vi "ProgBar_UI.vi"() -> ()   [LabVIEW 2020]
doc: ",,,,,,,,,,,,,,,,,,,,,,,,,,,,,,,,,,,,,,,,,,,,,,,,,,,,,,,,,,,,,,,,,,,,,,,,,,,,,,,,,,,,,,,,,,,,,,,,,,,,,,,,,,,,,,,,,,,,,,,,,,,,,,,,,,,,,,,,,,,,,,,,"
uses:
  controls/ProgBar_Element.ctl
  controls/System_Custom/Cancel.ctl
  controls/ProgBar_Msg.ctl
  <vilib>/Utility/miscctls.llb/LVRectTypeDef.ctl
  <vilib>/Utility/miscctls.llb/LVPositionTypeDef.ctl
panel:
  out "Current_Prgrs":T3(array[cluster]) {"ProgBar_El"."Curr Digital" format="%#_7g"; "ProgBar_El"."Slide Value" scale=0.0..100.0}
  in  "Display":T1[](array[typedef]) {"Curr Digital" format="%#_7g"; "Slide Value" scale=0.0..100.0}
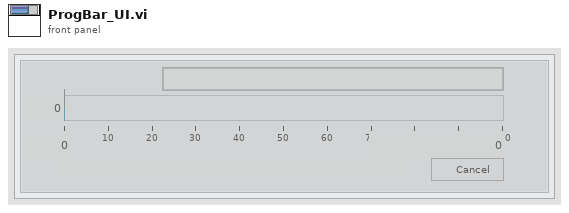
[diagram p1: front panel]
types:
  T1 = typedef "ProgBar_Element.ctl" = cluster{"Label":string, "Slide Value":i32, "Max":dbl, "Curr Digital":dbl, "Min":dbl, "State Info":string, "Cancel":T2}
  T2 = typedef "Cancel.ctl" = bool
  T3 = cluster{"Progress Queue Name":string, "ProgBar_El":T1}[]
  T4 = typedef "ProgBar_Msg.ctl" = cluster{"Que_Name":string, "Label":string, "Max Number of Iterations":i32, "Current Iteration ":i32, "State Info(Optional)":string, "Stop":bool}
  T5 = enum32{"Invalid", "Default", "Floating", "Floating/Auto-Hide", "Modal"}
  T6 = typedef "LVPositionTypeDef.ctl" = cluster{"Left":i32, "Top":i32}
  T7 = typedef "LVRectTypeDef.ctl" = cluster{"Left":i16, "Top":i16, "Right":i16, "Bottom":i16}
  T8 = typedef "LVBoundsTypeDef.ctl" = cluster{"Width":u32, "Height":u32}
  T9 = cluster{"Label":bool, "Slide Value":bool, "Max":bool, "Curr Digital":bool, "Min":bool, "State Info":bool, "Cancel":T2}[]
  T10 = cluster{"Progress Queue Name":string, "ProgBar_El":T1}
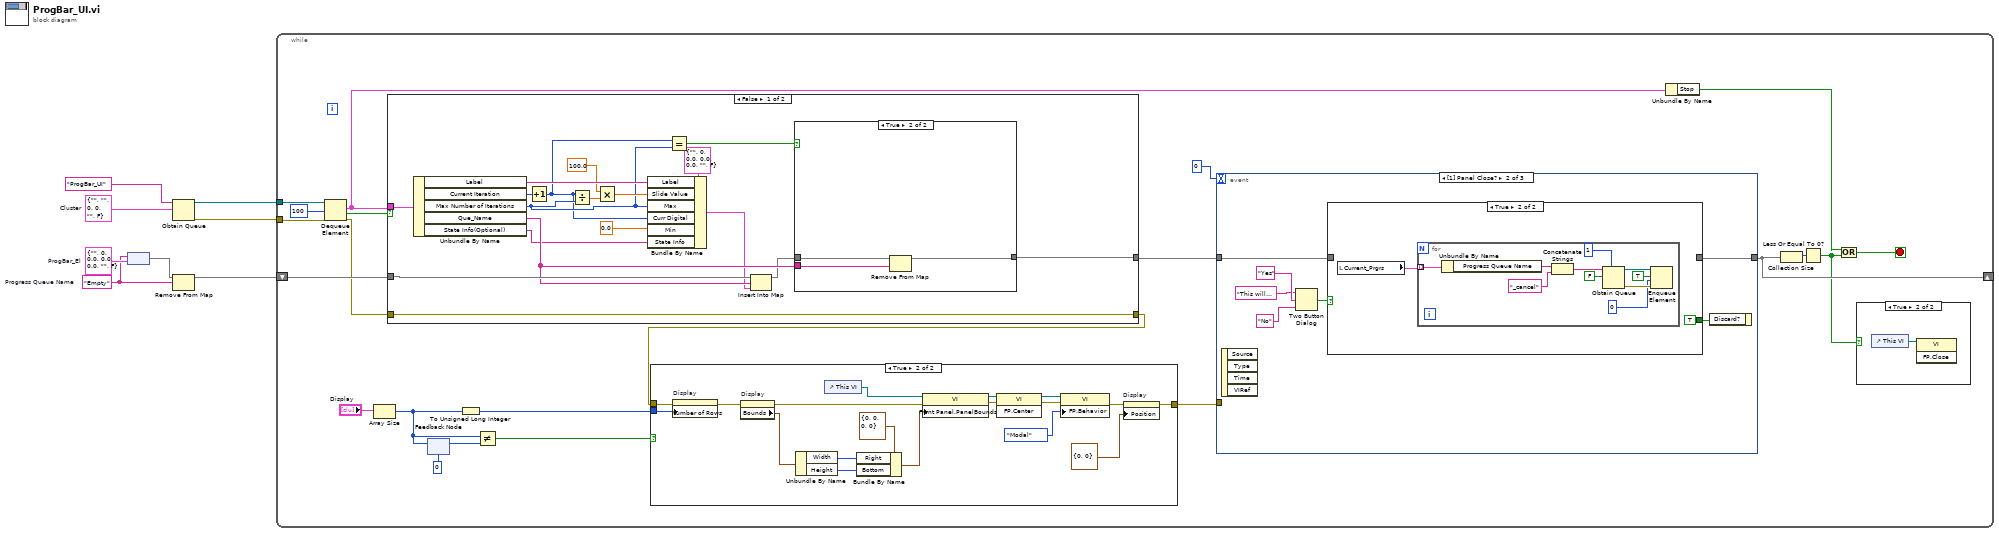
[diagram p0: block diagram]
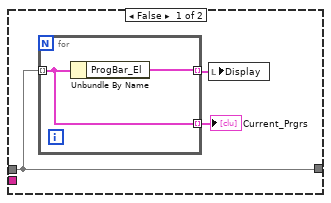
[diagram p2: hidden frame]
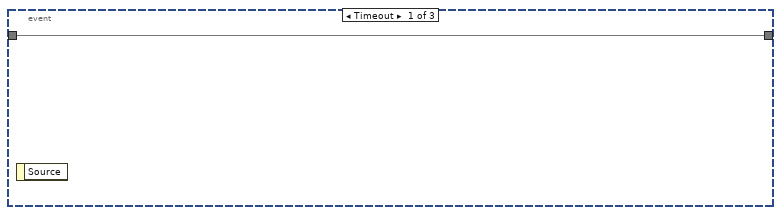
[diagram p5: hidden frame]
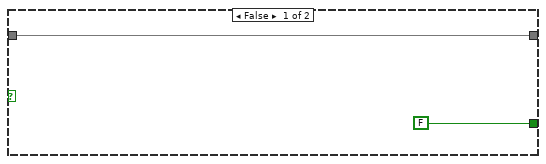
[diagram p6: hidden frame]
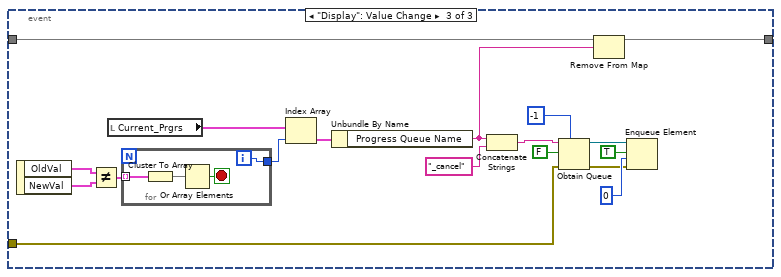
[diagram p7: hidden frame]
diagram:
  w6 = "Empty"  # Progress Queue Name
  w7 = T1 {"Label"="", "Slide Value"=0, "Max"=0.0, "Curr Digital"=0.0, "Min"=0.0, "State Info"="", "Cancel"=FALSE}  # ProgBar_El
  w4 = T4 {"Que_Name"="", "Label"="", "Max Number of Iterations"=0, "Current Iteration "=0, "State Info(Optional)"="", "Stop"=FALSE}  # Cluster
  n1 = node(w6, w7) -> (w5:map{string, T1})
  n2 = Obtain Queue(name (unnamed)="ProgBar_UI" ("Progress Queue Name"), element data type=w4) -> (queue out=w1:refnum<queue>, error out=w2:errorcluster)  [unwired: 3 in, 1 out]
  n3 = Remove From Map(10:w6, 11:w5) -> (3:w3:map{string, T1})  [unwired: 2 out]
  n4 = while {
    tunnel: w1 -> [w30]
    shift-right: [w17] -> _
    shift-left: w3 -> [w29]
    tunnel: w2 -> [w22]
    stop <- w10 stop-if-true
    n5 = Dequeue Element(queue=w30, timeout in ms (-1)=100, error in (no error)=w22) -> (element=w12:T4, timed out?=w25:bool, error out=w24:errorcluster)  [unwired: 1 out]
    n6 = Array Size(array="Display") -> (size(s)=w15:i32)
    n7 = case shown="False" w25 {
      tunnel: w12 -> [w48 _]
      tunnel: w29 -> [w45 w58]
      tunnel: [w35 w58] -> w16
      tunnel: [w44 w57] -> w14
      tunnel: w24 -> [w44 w57]
      frame False {
        n8 = Unbundle By Name(w48) -> ("Label"=w46:string, "Current Iteration"=w32:i32, "Max Number of Iterations"=w33:i32, "Que_Name"=w38:string, "State Info(Optional)"=w37:string)
        n9 = Increment(x=w32) -> (x+1=w31:i32)
        n10 = Divide(x=w31, y=w33) -> (x/y=w41:dbl)
        n11 = Multiply(x=100.0 ("y"), y=w41) -> (x*y=w40:dbl)
        n12 = Bundle By Name(cluster=T1 {"Label"="", "Slide Value"=0, "Max"=0.0, "Curr Digital"=0.0, "Min"=0.0, "State Info"="", "Cancel"=FALSE} ("Cluster 2"), "Label"=w46, "Slide Value"=w40, "Max"=w33, "Curr Digital"=w31, "Min"=0.0, "State Info"=w37) -> (w36:T1)
        n13 = Equal?(x=w31, y=w33) -> (x = y?=w43:bool)
        n14 = Insert Into Map(map in=w45, key=w38, value=w36) -> (map out=w34:map{string, T1})  [unwired: 2 out]
        n15 = case shown="True" w43 {
          tunnel: w38 -> [_ w55]
          tunnel: w34 -> [w49 w56]
          tunnel: [w49 w54] -> w35
          frame False {
            n16 = for {
              tunnel: [w53] -> w50 mode=indexing
              tunnel: w49 -> [w52] mode=indexing
              tunnel: [w52] -> w51 mode=indexing
              n17 = Unbundle By Name(w52) -> ("ProgBar_El"=w53:T1)
            }
            "Current_Prgrs" <- w51
            n18 = local write "Display"(w50) -> ()
          }
          frame True {
            n19 = Remove From Map(10:w55, 11:w56) -> (3:w54:map{string, T1})  [unwired: 2 out]
          }
        }
      }
      frame True {
      }
    }
    n20 = feedback #1(0) -> (w21:i32)
    n21 = feedback-in #1(w15) -> ()
    n22 = To Unsigned Long Integer(number=w15) -> (unsigned 32bit integer=w23:u32)
    n23 = Not Equal?(x=w15, y=w21) -> (x != y?=w20:bool)
    n24 = case shown="True" w20 {
      tunnel: w23 -> [_ w74]
      tunnel: w14 -> [w59 w73]
      tunnel: [w59 w67] -> w19
      frame False {
      }
      frame True {
        n25 = property on="Display" class="Arr (strict)"(error in=w73, "Number of Rows"=w74) -> (error out=w65:errorcluster)  [unwired: 1 in, 1 out]
        n26 = property on="Display" class="Arr (strict)"(error in=w65) -> (error out=w75:errorcluster, "Bounds"=w77:T8)  [unwired: 1 in, 1 out]
        n27 = Unbundle By Name(w77) -> ("Width"=w72:u32, "Height"=w71:u32)
        n28 = control-ref of="This VI"() -> (w64:refnum<vi>)
        n29 = Bundle By Name(cluster=T7 {"Left"=0, "Top"=0, "Right"=0, "Bottom"=0} ("Front Panel Window:Window Bounds"), "Right"=w72, "Bottom"=w71) -> (w76:T7)
        n30 = property class="VI"(reference=w64, error in=w75, "Front Panel.PanelBounds"=w76) -> (reference out=w69:refnum<vi>, error out=w68:errorcluster)
        n31 = invoke class="VI" method="FP.Center"(reference=w69, error in=w68) -> (reference out=w60:refnum<vi>, error out=w63:errorcluster)  [unwired: 1 in, 1 out]
        n32 = property class="VI"(reference=w60, error in=w63, "FP.Behavior"=T5."Modal" ("Front Panel Window:Behavior")) -> (error out=w61:errorcluster)  [unwired: 1 out]
        n33 = property on="Display" class="Arr (strict)"(error in=w61, "Position"=T6 {"Left"=0, "Top"=0}) -> (error out=w67:errorcluster)  [unwired: 1 in, 1 out]
      }
    }
    n34 = event shown="[1] Panel Close?" {
      selector: _ -> [_ _ _]
      dyn-events: _ -> [_ _ _]
      timeout: 0 -> [_ _ _]
      tunnel: [w78 w80 w105] -> w17
      tunnel: w16 -> [w78 w81 w102]
      tunnel: w19 -> [_ _ w101]
      event Timeout {
        n35 = event-data() -> ()  [unwired: 1 in, 1 out]
      }
      event Panel Close? {
        n36 = event-data() -> ()  [unwired: 1 in, 4 out]
        n37 = Two Button Dialog(message="This will cancel all ongoing processes. Do you want to proceed?", 1:"No" ("F button name (\"Cancel\")"), 2:"Yes" ("T button name (\"OK\")")) -> (T button?=w82:bool)
        n38 = case shown="True" w82 {
          tunnel: [FALSE ("Discard?") TRUE ("Discard?")] -> w79
          tunnel: w81 -> [w86 _]
          tunnel: [w86 _] -> w80
          frame False {
          }
          frame True {
            n39 = local read "Current_Prgrs"() -> (w89:T3)
            n40 = for {
              tunnel: w89 -> [w90] mode=indexing
              n41 = Unbundle By Name(w90) -> ("Progress Queue Name"=w97:string)
              n42 = Concatenate Strings(w97, "_cancel" ("string")) -> (w99:string)
              n43 = Obtain Queue(max queue size (-1, unlimited)=1, name (unnamed)=w99, element data type=FALSE ("element")) -> (queue out=w98:refnum<queue>, error out=w96:errorcluster)  [unwired: 2 in, 1 out]
              n44 = Enqueue Element(queue=w98, element=TRUE, timeout in ms (-1)=0, error in (no error)=w96) -> ()  [unwired: 3 out]
            }
          }
        }
        n45 = event-data("Discard?"=w79) -> ()  [unwired: 1 in, 1 out]
      }
      event "Display": Value Change {
        n46 = event-data() -> ("OldVal"=w117:T1[], "NewVal"=w116:T1[])  [unwired: 1 in]
        n47 = Not Equal?(x=w117, y=w116) -> (x != y?=w115:T9)
        n48 = local read "Current_Prgrs"() -> (w114:T3)
        n49 = for {
          tunnel: w115 -> [w121] mode=indexing
          tunnel: [w118] -> w113
          i -> [w118]
          stop <- w119 stop-if-true
          n50 = Cluster To Array(cluster=w121) -> (array=w120:T2[])
          n51 = Or Array Elements(Boolean array=w120) -> (logical OR=w119:bool)
        }
        n52 = Index Array(array=w114, index=w113) -> (element=w112:T10)
        n53 = Unbundle By Name(w112) -> ("Progress Queue Name"=w104:string)
        n54 = Concatenate Strings(w104, "_cancel" ("string")) -> (w110:string)
        n55 = Obtain Queue(max queue size (-1, unlimited)=-1, name (unnamed)=w110, element data type=FALSE ("element"), error in (no error)=w101) -> (queue out=w109:refnum<queue>, error out=w100:errorcluster)  [unwired: 1 in, 1 out]
        n56 = Remove From Map(10:w104, 11:w102) -> (3:w105:map{string, T1})  [unwired: 2 out]
        n57 = Enqueue Element(queue=w109, element=TRUE, timeout in ms (-1)=0, error in (no error)=w100) -> ()  [unwired: 3 out]
      }
    }
    n58 = Unbundle By Name(w12) -> ("Stop"=w11:bool)
    n59 = Collection Size(1:w17) -> (0:w28:i32)
    n60 = Less Or Equal To 0?(x=w28) -> (x <= 0?=w9:bool)
    n61 = Or(x=w11, y=w9) -> (x .or. y?=w10:bool)
    n62 = case shown="True" w9 {
      frame False {
      }
      frame True {
        n63 = control-ref of="This VI"() -> (w122:refnum<vi>)
        n64 = invoke class="VI" method="FP.Close"(reference=w122) -> ()  [unwired: 2 in, 3 out]
      }
    }
  }
